vi "graddphelper.vi"(10 "dxda,dyda":dbl[][](array[numeric]), 11 "dfdx,dfdy":dbl[][](array[numeric])) -> (2 "dfda":dbl[](array[numeric]))   [LabVIEW 2017]
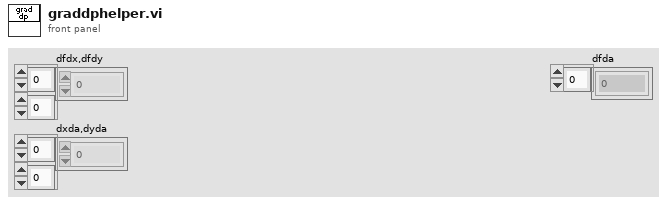
[diagram p1: front panel]
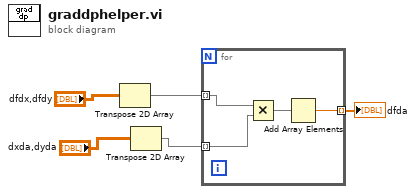
[diagram p0: block diagram]
diagram:
  n1 = Transpose 2D Array(2D array="dfdx,dfdy") -> (transposed array=w2:dbl[][])
  n2 = Transpose 2D Array(2D array="dxda,dyda") -> (transposed array=w3:dbl[][])
  n3 = for {
    tunnel: w2 -> [w9] mode=indexing
    tunnel: w3 -> [w8] mode=indexing
    tunnel: [w6] -> w1 mode=indexing
    n4 = Multiply(x=w9, y=w8) -> (x*y=w7:dbl[])
    n5 = Add Array Elements(numeric array=w7) -> (sum=w6:dbl)
  }
  "dfda" <- w1
